vi "Get CPU Hardware Info.vi"(8 "error in (no error)":errorcluster, 11 "Hardware Info in":refnum<class "Hardware Info.lvclass">) -> (0 "error out":errorcluster, 2 "CPU Info":refnum<class "CPU Hardware Info.lvclass">, 3 "Hardware Info out":refnum<class "Hardware Info.lvclass">)   [LabVIEW 2017, in "Data Sharing Framework Core.lvlib" / "Data Sharing Framework Engine.lvlib" / "Hardware Info.lvclass"]
uses:
  Hardware Info.lvclass
  CPU Hardware Info/CPU Hardware Info.lvclass
  Hardware Info.lvclass/Hardware Info.ctl
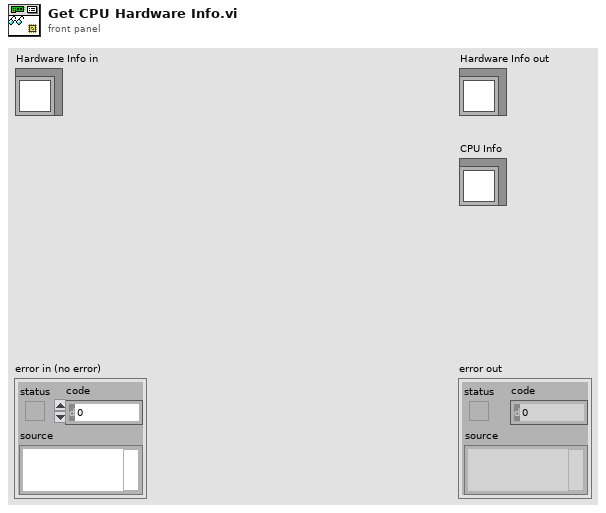
[diagram p1: front panel]
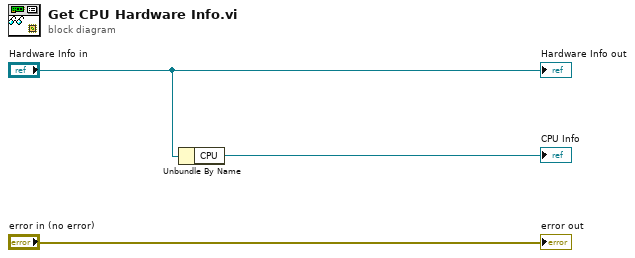
[diagram p0: block diagram]
diagram:
  n1 = Unbundle By Name("Hardware Info in") -> ("CPU"=→"CPU Info":refnum<class "CPU Hardware Info.lvclass">)
  "error out" <- "error in (no error)"
  "Hardware Info out" <- "Hardware Info in"
